vi "DP-Artifact Rejection.vi"(5 "DataAcq":T1, 7 "Reject Ref":T2, 9 "DP Freqs":T3, 11 "Magnitude (Vrms)":dbl[](array[numeric])) -> (3 "Reject?":bool)   [LabVIEW 2020]
uses:
  Typedefs/DP-Freqs.ctl
  Typedefs/DP-Rejection Settings Refnum.ctl
  Typedefs/DP-Rejection Settings.ctl
  Typedefs/DP-DataAcq.ctl
  epl-vi-lib/Utility VIs/Math VIs/Linear to dB (scalar).vi
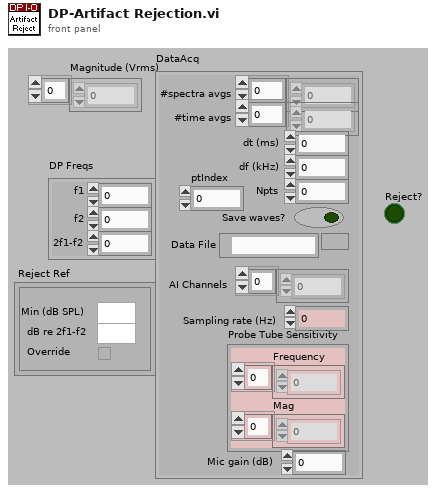
[diagram p1: front panel]
types:
  T1 = typedef "DP-DataAcq.ctl" = cluster{"#spectra avgs":i32[], "#time avgs":i32[], "dt (ms)":dbl, "df (kHz)":dbl, "Npts":i32, "Save waves?":bool, "Data File":path, "AI Channels":u16[], "Sampling rate (Hz)":dbl, "Probe Tube Sensitivity":cluster{"Frequency":dbl[], "Mag":dbl[]}, "Mic gain (dB)":dbl, "ptIndex":i32}
  T2 = typedef "DP-Rejection Settings Refnum.ctl" = refnum<vi>
  T3 = typedef "DP-Freqs.ctl" = cluster{"f1":dbl, "f2":dbl, "2f1-f2":dbl}
  T4 = typedef "DP-Rejection Settings.ctl" = cluster{"Override":bool, "dB re 2f1-f2":dbl, "Min (dB SPL)":dbl}
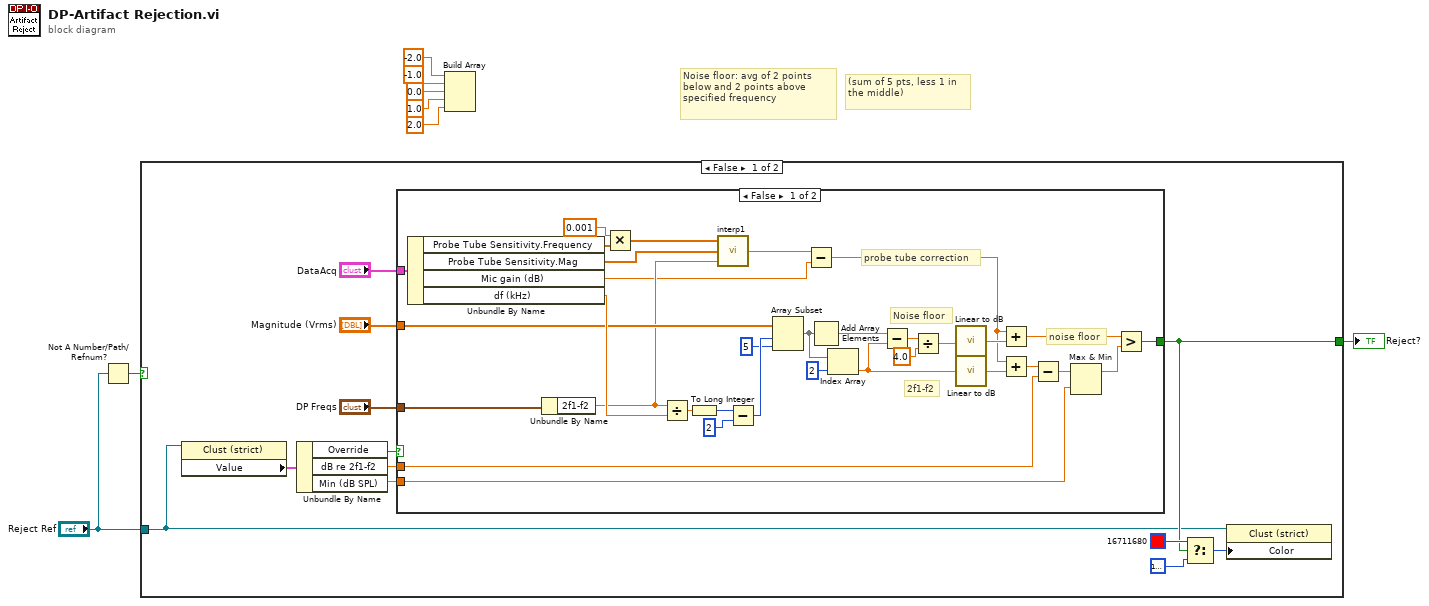
[diagram p0: block diagram]
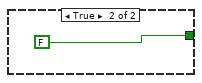
[diagram p2: hidden frame]
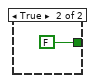
[diagram p3: hidden frame]
diagram:
  # "(sum of 5 pts, less 1 in the middle)"
  # "Noise floor: avg of 2 points\nbelow and 2 points above specified frequency"
  n1 = Not A Number/Path/Refnum?(number/path/refnum="Reject Ref") -> (NaN/Path/Refnum?=w2:bool)
  n2 = case shown="False" w2 {
    tunnel: [w10 FALSE] -> w8
    tunnel: "Reject Ref" -> [w9 _]
    frame False {
      n3 = property class="Clust (strict)"(reference=w9) -> ("Value"=w16:T4)  [unwired: 1 in, 2 out]
      n4 = Unbundle By Name(w16) -> ("Override"=w18:bool, "dB re 2f1-f2"=w17:dbl, "Min (dB SPL)"=w14:dbl)
      n5 = case shown="False" w18 {
        tunnel: "DP Freqs" -> [w52 _]
        tunnel: "Magnitude (Vrms)" -> [w37 _]
        tunnel: [w44 FALSE] -> w10
        tunnel: w17 -> [w25 _]
        tunnel: "DataAcq" -> [w43 _]
        tunnel: w14 -> [w23 _]
        frame False {
          # "noise floor"
          # "2f1-f2"
          # "Noise floor"
          # "probe tube correction"
          n6 = Unbundle By Name(w43) -> ("Probe Tube Sensitivity.Frequency"=w41:dbl[], "Probe Tube Sensitivity.Mag"=w38:dbl[], "Mic gain (dB)"=w30:dbl, "df (kHz)"=w42:dbl)
          n7 = Unbundle By Name(w52) -> ("2f1-f2"=w34:dbl)
          n8 = Multiply(x=0.001, y=w41) -> (x*y=w39:dbl[])
          n9 = Divide(x=w34, y=w42) -> (x/y=w53:dbl)
          n10 = To Long Integer(number=w53) -> (32bit integer=w51:i32)
          n11 = call "interp1.vi"("X"=w39, "Y"=w38, "U"=w34) -> ("V"=w31:dbl)  [unwired: 2 in]
          n12 = Subtract(x=w51, y=2) -> (x-y=w49:i32)
          n13 = Array Subset(array=w37, index=w49, length=5) -> (w36:dbl[])
          n14 = Subtract(x=w31, y=w30) -> (x-y=w28:dbl)
          n15 = Add Array Elements(numeric array=w36) -> (sum=w45:dbl)
          n16 = Index Array(array=w36, index=2) -> (element=w32:dbl)
          n17 = Subtract(x=w45, y=w32) -> (x-y=w47:dbl)
          n18 = Divide(x=w47, y=4.0) -> (x/y=w33:dbl)
          n19 = call-poly "Linear to dB.vi"("Linear"=w33) -> ("dB"=w29:dbl)
          n20 = call-poly "Linear to dB.vi"("Linear"=w32) -> ("dB"=w27:dbl)
          n21 = Add(x=w28, y=w29) -> (x+y=w21:dbl)
          n22 = Add(x=w28, y=w27) -> (x+y=w26:dbl)
          n23 = Subtract(x=w26, y=w25) -> (x-y=w24:dbl)
          n24 = Max & Min(x=w24, y=w23) -> (max(x,y)=w22:dbl)  [unwired: 1 out]
          n25 = Greater?(x=w21, y=w22) -> (0:w44:bool)
        }
        frame True {
        }
      }
      n26 = Select(t=u32 16711680, s=w10, f=u32 16777238) -> (s? t:f=w11:u32)
      n27 = property class="Clust (strict)"(reference=w9, "Color"=w11) -> ()  [unwired: 1 in, 2 out]
    }
    frame True {
    }
  }
  "Reject?" <- w8
  n28 = Build Array(-2.0, -1.0, 0.0, 1.0, 2.0) -> ()  [unwired: 1 out]
